vi "COMTRADE Read Private Inf (1 Entry).vi"(7 "entry name":string, 8 "error in (no error)":errorcluster, 9 "section name":string, 10 "manufacturer name":string, 11 "task in":T1={"file refnums"=[], "Data Object"=refnum, "config info"={"station_name"="", "rec_dev_id"="", "rev_year"=1999.0, "TT"=0, "##A"=0, "##D"=0, "analog channel info"=[], "status channel info"=[], "lf"=50.0, "nrates"=0, "samp info"=[], "initial timestamp"=timestamp(0 s since 1904-01-01), "trigger timestamp"=timestamp(0 s since 1904-01-01), "ft"=enum."Binary", "timemult"=1.0}, "public inf content"={"Source"="", "Record Type"=enum."Unknown", "Phase ID"="", "Event Description"="", "Device ID"="", "Distance of Fault"=-1.0, "Distance Unit"=enum."Miles", "Max_Current"=inf, "Min_Current"=-inf, "Max_Voltage"=inf, "Min_Voltage"=-inf, "EventNoteCount"=0, "Event Information"=[]}, "private inf content"=[], "internal buffers"={"start index"=1, "config to public inf"=enum."disabled", "static config info"="", "static file_des record inf"="", "static file_des channel inf"="", "public inf"="", "private inf"=""}} {"public inf content"."Event Information"."min sample number" max=9999999999; "public inf content"."Event Information"."max sample number" max=9999999999; "config info"."nrates" max=999; "config info"."status channel info"."Dn" min=1 max=999999; "config info"."analog channel info"."An" min=1 max=999999; "config info"."trigger timestamp" format="%<%H:%M:%S%6u\n%d/%m/%Y>T"; "config info"."initial timestamp" format="%<%H:%M:%S%6u\n%d/%m/%Y>T"; "config info"."##D" max=999999; "config info"."##A" max=999999; "config info"."TT" min=1 max=999999; "config info"."rev_year" min=1999.0 max=1999.0}) -> (0 "error out":errorcluster, 1 "entry value":string, 3 "task out":T1={"file refnums"=[], "Data Object"=refnum, "config info"={"station_name"="", "rec_dev_id"="", "rev_year"=1999.0, "TT"=0, "##A"=0, "##D"=0, "analog channel info"=[], "status channel info"=[], "lf"=50.0, "nrates"=0, "samp info"=[], "initial timestamp"=timestamp(0 s since 1904-01-01), "trigger timestamp"=timestamp(0 s since 1904-01-01), "ft"=enum."Binary", "timemult"=1.0}, "public inf content"={"Source"="", "Record Type"=enum."Unknown", "Phase ID"="", "Event Description"="", "Device ID"="", "Distance of Fault"=-1.0, "Distance Unit"=enum."Miles", "Max_Current"=inf, "Min_Current"=-inf, "Max_Voltage"=inf, "Min_Voltage"=-inf, "EventNoteCount"=0, "Event Information"=[]}, "private inf content"=[], "internal buffers"={"start index"=1, "config to public inf"=enum."disabled", "static config info"="", "static file_des record inf"="", "static file_des channel inf"="", "public inf"="", "private inf"=""}} {"public inf content"."Event Information"."min sample number" max=9999999999; "public inf content"."Event Information"."max sample number" max=9999999999; "config info"."nrates" max=999; "config info"."status channel info"."Dn" min=1 max=999999; "config info"."analog channel info"."An" min=1 max=999999; "config info"."trigger timestamp" format="%<%H:%M:%S%6u\n%d/%m/%Y>T"; "config info"."initial timestamp" format="%<%H:%M:%S%6u\n%d/%m/%Y>T"; "config info"."##D" max=999999; "config info"."##A" max=999999; "config info"."TT" min=1 max=999999; "config info"."rev_year" min=1999.0 max=1999.0}, 4 "entry found?":bool)   [LabVIEW 2013, in "NI_EP_COMTRADE.lvlib"]
doc: "Reads information from the private sections of the optionally specified .inf file. You must set <B>open mode</B> to Open (read only) in the COMTRADE Open VI to open the .inf file. Otherwise this VI returns an error."
uses:
  <vilib>/addons/Electrical Power/File IO/NI_EP_COMTRADE.lvlib
  <vilib>/addons/Electrical Power/File IO/COMTRADE/typedefs/ep_Task.ctl
  <vilib>/addons/Electrical Power/File IO/COMTRADE/typedefs/ep_Config Info.ctl
  <vilib>/addons/Electrical Power/File IO/COMTRADE/typedefs/ep_Analog Channel Info.ctl
  <vilib>/addons/Electrical Power/File IO/COMTRADE/typedefs/ep_Status Channel Info.ctl
  <vilib>/addons/Electrical Power/File IO/COMTRADE/typedefs/ep_File Format.ctl
  <vilib>/addons/Electrical Power/File IO/COMTRADE/typedefs/ep_Public Inf Content.ctl
  <vilib>/addons/Electrical Power/File IO/COMTRADE/typedefs/ep_Public Event Inf.ctl
  <vilib>/addons/Electrical Power/File IO/COMTRADE/typedefs/ep_Private Inf Content.ctl
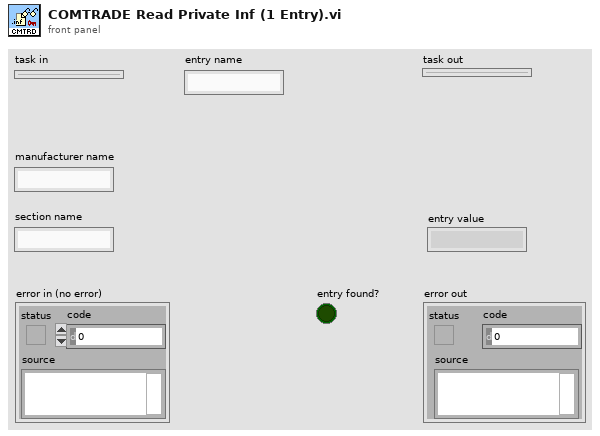
[diagram p1: front panel]
types:
  T1 = typedef "NI_EP_COMTRADE.lvlib/ep_Task.ctl" = cluster{"file refnums":refnum<file>[], "Data Object":refnum<k20>, "config info":T2, "public inf content":T6, "private inf content":T8, "internal buffers":cluster{"start index":u32, "config to public inf":enum16{"disabled", "enabled", "buffered"}, "static config info":string, "static file_des record inf":string, "static file_des channel inf":string, "public inf":string, "private inf":string}}
  T2 = typedef "NI_EP_COMTRADE.lvlib/ep_Config Info.ctl" = cluster{"station_name":string, "rec_dev_id":string, "rev_year":dbl, "TT":u32, "##A":u32, "##D":u32, "analog channel info":T3[], "status channel info":T4[], "lf":sgl, "nrates":u16, "samp info":cluster{"samp":sgl, "endsamp":u32}[], "initial timestamp":timestamp, "trigger timestamp":timestamp, "ft":T5, "timemult":sgl}
  T3 = typedef "NI_EP_COMTRADE.lvlib/ep_Analog Channel Info.ctl" = cluster{"An":u32, "ch_id":string, "ph":string, "ccbm":string, "uu":string, "a":sgl, "b":sgl, "skew":sgl, "min":i32, "max":i32, "primary":sgl, "secondary":sgl, "PS":enum16{"P", "S"}}
  T4 = typedef "NI_EP_COMTRADE.lvlib/ep_Status Channel Info.ctl" = cluster{"Dn":u32, "ch_id":string, "ph":string, "ccbm":string, "Y":bool}
  T5 = typedef "NI_EP_COMTRADE.lvlib/ep_File Format.ctl" = enum16{"ASCII", "Binary"}
  T6 = typedef "NI_EP_COMTRADE.lvlib/ep_Public Inf Content.ctl" = cluster{"Source":string, "Record Type":enum16{"Fault", "Unknown", "Misoperation", "Close", "Trip", "Reclose", "Power swing", "Simulation"}, "Phase ID":string, "Event Description":string, "Device ID":string, "Distance of Fault":dbl, "Distance Unit":enum16{"Miles", "Kilometers", "Percent of line", "Percent of setting", "Ohms"}, "Max_Current":dbl, "Min_Current":dbl, "Max_Voltage":dbl, "Min_Voltage":dbl, "EventNoteCount":u32, "Event Information":T7[]}
  T7 = typedef "NI_EP_COMTRADE.lvlib/ep_Public Event Inf.ctl" = cluster{"channel number":u32, "max value":dbl, "min value":dbl, "max sample number":u64, "min sample number":u64, "max sample text":string[], "min sample text":string[]}
  T8 = typedef "NI_EP_COMTRADE.lvlib/ep_Private Inf Content.ctl" = cluster{"Section Header":string, "Entry Names":string[], "Entry Values":string[]}[]
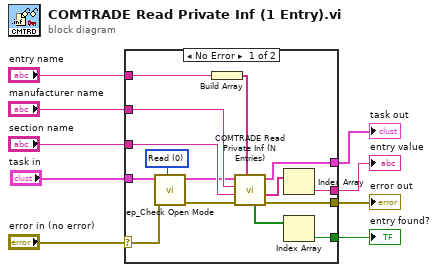
[diagram p0: block diagram]
diagram:
  n1 = case shown="No Error" "error in (no error)" {
    selector: "error in (no error)" -> [w11 w25]
    tunnel: "task in" -> [w12 w26]
    tunnel: [w24 w26] -> w7
    tunnel: [w19 w25] -> w6
    tunnel: "entry name" -> [w23 _]
    tunnel: "manufacturer name" -> [w21 _]
    tunnel: "section name" -> [w20 _]
    tunnel: [w18 _] -> w1
    tunnel: [w17 _] -> w2
    frame No Error {
      w14 = u16 0 items=["Read", "Write"] ("file type")
      n2 = call <vilib>:"ep_Check Open Mode.vi"("expected mode"=w14, "error in (no error)"=w11, "task in"=w12) -> ("error out"=w10:errorcluster, "task out"=w13:T1)  [unwired: 7 in]
      n3 = Build Array(w23) -> (w22:string[])
      n4 = call <vilib>:"COMTRADE Read Private Inf (N Entries).vi"("entry names"=w22, "error in (no error)"=w10, "section name"=w20, "manufacturer name"=w21, "task in"=w13) -> ("error out"=w19:errorcluster, "entry values"=w15:string[], "task out"=w24:T1, "entries found?"=w16:bool[])  [unwired: 3 in]
      n5 = Index Array(array=w15) -> (element=w18:string)  [unwired: 1 in]
      n6 = Index Array(array=w16) -> (element=w17:bool)  [unwired: 1 in]
    }
    frame Error {
    }
  }
  "task out" <- w7
  "error out" <- w6
  "entry found?" <- w2
  "entry value" <- w1
